vi "CombiningVIs_EV3.vi"() -> ()   [LabVIEW 2012]
uses:
  <vilib>/NXT/Subs/MotorOutput.ctl
  SubVIs/LVPresent_Globals.vi
panel:
  in  "Run":bool
  in  "Open":bool
  # "Combining VIs\n\nYou can add multiple VIs together on the diagram - and if you wire them together, the pink line defines the order in which things execute.  Wires contain data, and the second VI on a string cannot run until the first is complete and puts data on the pink wire.  If there were no wire, both VIs would run at the same time.  Click the Run button to try out the program. Then use the Open button to open the program in LabVIEW, and play around with the code."
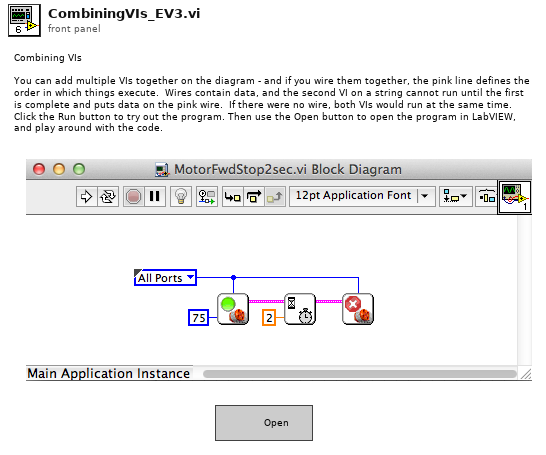
[diagram p1: front panel]
types:
  T1 = typedef "MotorOutput.ctl" = u8
  T2 = typedef "LVHSConnector.ctl" = refnum<class "BrickReference.lvclass">
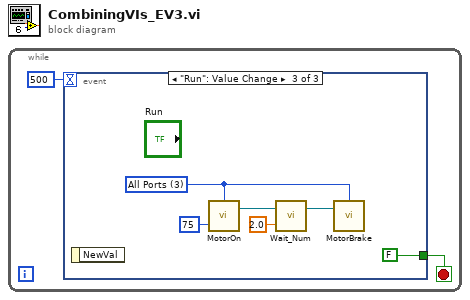
[diagram p0: block diagram]
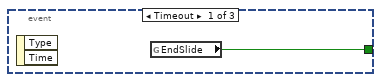
[diagram p2: hidden frame]
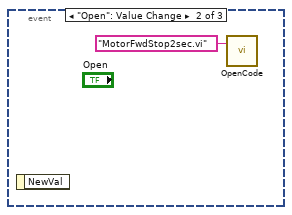
[diagram p3: hidden frame]
diagram:
  n1 = while {
    stop <- w2 stop-if-true
    n2 = event shown="[2] \"Run\": Value Change" {
      selector: _ -> [_ _ _]
      dyn-events: _ -> [_ _ _]
      timeout: 500 -> [_ _ _]
      tunnel: [w3 _ FALSE] -> w2
      event Timeout {
        n3 = event-data() -> ()  [unwired: 1 in, 2 out]
        n4 = global read "LVPresent_Globals.vi" "EndSlide"() -> (w3:bool)
      }
      event "Open": Value Change {
        n5 = event-data() -> ()  [unwired: 1 in, 1 out]
        n6 = call "OpenCode.vi"("Code name"="MotorFwdStop2sec.vi") -> ()  [unwired: 3 in]
      }
      event "Run": Value Change {
        w6 = T1 3 items=["Port A"=0, "Port B"=1, "Port C"=2, "Ports A & B"=4, "Ports A & C"=5, "Ports B & C"=6, "All Ports"=3] ("Output Port (All Ports)")
        n7 = event-data() -> ()  [unwired: 1 in, 1 out]
        n8 = call <vilib>:"MotorOn.vi"("Power (75)"=75, "Output Port (All Ports)"=w6) -> ("NXT/EV3"=w10:T2)  [unwired: 2 in]
        n9 = call <vilib>:"Wait_Num.vi"("Time (1 sec)"=sgl 2.0, "NXT/EV3"=w10) -> ("NXT/EV3"=w9:T2)  [unwired: 2 in]
        n10 = call <vilib>:"MotorBrake.vi"("NXT/EV3"=w9, "Port (All Ports)"=w6) -> ()  [unwired: 2 in, 1 out]
      }
    }
  }
